vi "Get Section.vi"(10 "section":string, 11 "element":T1) -> (0 "section exists?":bool, 2 "section data":T2, 3 "element out":T1, 4 "section index":i32)   [LabVIEW 2020, in "NI_LVConfig.lvlib"]
uses:
  NI_LVConfig.lvlib
  Section.ctl
  <vilib>/Utility/config.llb/Config Data.ctl
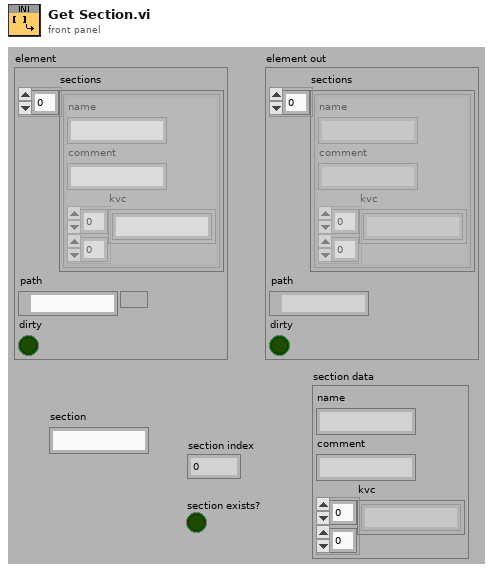
[diagram p1: front panel]
types:
  T1 = typedef "NI_LVConfig.lvlib/Config Data.ctl" = cluster{"sections":T2[], "path":path, "dirty":bool}
  T2 = typedef "NI_LVConfig.lvlib/Section.ctl" = cluster{"name":string, "comment":string, "kvc":string[][]}
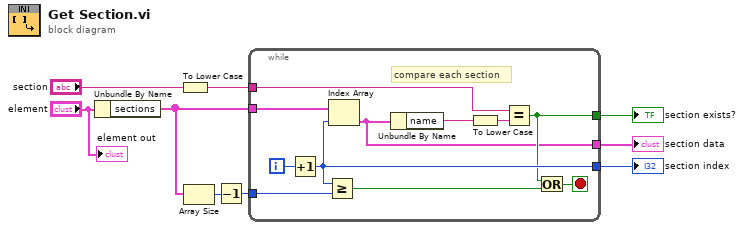
[diagram p0: block diagram]
diagram:
  n1 = Unbundle By Name("element") -> ("sections"=w6:T2[])
  n2 = To Lower Case(string="section") -> (all lower case string=w2:string)
  n3 = Array Size(array=w6) -> (size(s)=w5:i32)
  n4 = Decrement(x=w5) -> (x-1=w4:i32)
  n5 = while {
    tunnel: w2 -> [w20]
    tunnel: w6 -> [w19]
    tunnel: [w16] -> w9
    tunnel: [w14] -> w8
    tunnel: w4 -> [w15]
    tunnel: [w12] -> w7
    i -> [w17]
    stop <- w18 stop-if-true
    # "compare each section"
    n6 = Increment(x=w17) -> (x+1=w16:i32)
    n7 = Greater Or Equal?(x=w16, y=w15) -> (x >= y?=w13:bool)
    n8 = Index Array(array=w19, index=w16) -> (element=w12:T2)
    n9 = Unbundle By Name(w12) -> ("name"=w11:string)
    n10 = To Lower Case(string=w11) -> (all lower case string=w10:string)
    n11 = Equal?(x=w20, y=w10) -> (x = y?=w14:bool)
    n12 = Or(x=w14, y=w13) -> (x .or. y?=w18:bool)
  }
  "section index" <- w9
  "section exists?" <- w8
  "section data" <- w7
  "element out" <- "element"
